vi "Valid Replacement Target.vi"(8 "error in (no error)":errorcluster, 10 "missing paths":path[](array[path]), 11 "missing names":string[](array[string])) -> (0 "error out":errorcluster, 1 "valid replacement target":bool, 2 "missing path":path, 3 "missing name":string)   [LabVIEW 2020, in "MeasurementService Editor.lvlib"]
uses:
  MeasurementService Editor.lvlib
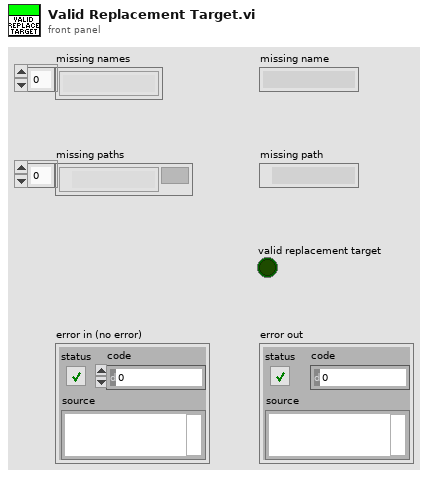
[diagram p1: front panel]
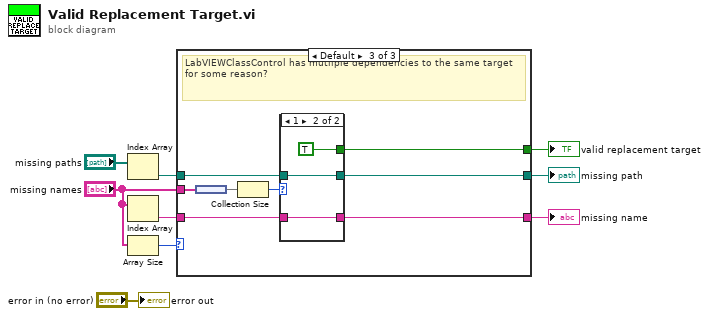
[diagram p0: block diagram]
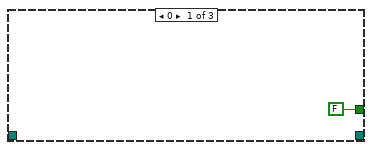
[diagram p2: hidden frame]
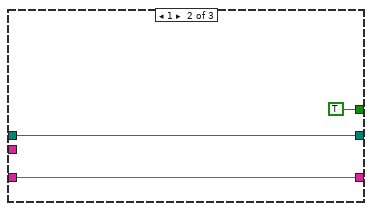
[diagram p3: hidden frame]
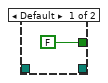
[diagram p4: hidden frame]
diagram:
  n1 = Index Array(array="missing paths") -> (element=w5:path)  [unwired: 1 in]
  n2 = Index Array(array="missing names") -> (element=w6:string)  [unwired: 1 in]
  n3 = Array Size(array="missing names") -> (size(s)=w7:i32)
  n4 = case shown="Default" w7 {
    tunnel: w6 -> [_ w13 w16]
    tunnel: w5 -> [_ w12 w14]
    tunnel: [_ w13 w17] -> w4
    tunnel: [_ w12 w15] -> w3
    tunnel: [FALSE TRUE w18] -> w2
    tunnel: "missing names" -> [_ _ w20]
    frame 0 {
    }
    frame 1 {
    }
    frame Default {
      # "LabVIEWClassControl has mutliple dependencies to the same target for some reason?"
      n5 = node(w20) -> (w21:set{string[]})
      n6 = Collection Size(1:w21) -> (0:w19:i32)
      n7 = case shown="1" w19 {
        tunnel: [FALSE TRUE] -> w18
        tunnel: [_ w24] -> w17
        tunnel: w16 -> [_ w24]
        tunnel: [_ w23] -> w15
        tunnel: w14 -> [_ w23]
        frame Default {
        }
        frame 1 {
        }
      }
    }
  }
  "missing path" <- w3
  "missing name" <- w4
  "valid replacement target" <- w2
  "error out" <- "error in (no error)"
